vi "dirty_detector.vi"(10 "dirty ROI":T1(array[cluster]), 11 "pixel2mil":dbl) -> (3 "area":dbl)   [LabVIEW 2017]
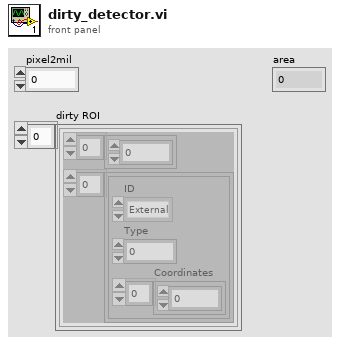
[diagram p1: front panel]
types:
  T1 = cluster{dbl[], cluster{"ID":enum32{"External", "Internal"}, "Type":u32, "Coordinates":i32[]}[]}[]
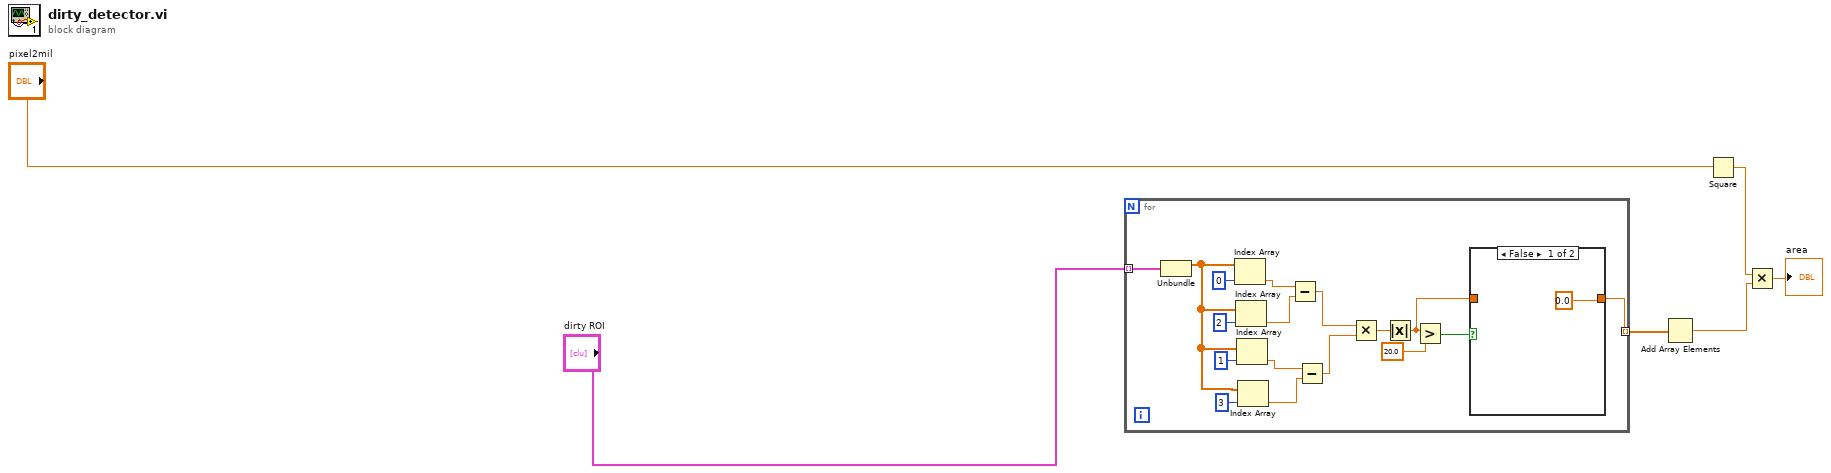
[diagram p0: block diagram]
diagram:
  n1 = for {
    tunnel: "dirty ROI" -> [w23] mode=indexing
    tunnel: [w8] -> w1 mode=indexing
    n2 = Unbundle(w23) -> (w18:dbl[])  [unwired: 1 out]
    n3 = Index Array(array=w18, index=0) -> (element=w17:dbl)
    n4 = Index Array(array=w18, index=2) -> (element=w16:dbl)
    n5 = Index Array(array=w18, index=1) -> (element=w15:dbl)
    n6 = Index Array(array=w18, index=3) -> (element=w14:dbl)
    n7 = Subtract(x=w17, y=w16) -> (x-y=w13:dbl)
    n8 = Subtract(x=w15, y=w14) -> (x-y=w12:dbl)
    n9 = Multiply(x=w13, y=w12) -> (x*y=w11:dbl)
    n10 = Absolute Value(x=w11) -> (abs(x)=w7:dbl)
    n11 = Greater?(x=w7, y=20.0) -> (0:w9:bool)
    n12 = case shown="False" w9 {
      tunnel: [0.0 ("y") w25] -> w8
      tunnel: w7 -> [_ w25]
      frame False {
      }
      frame True {
      }
    }
  }
  n13 = Add Array Elements(numeric array=w1) -> (sum=w5:dbl)
  n14 = Square(x="pixel2mil") -> (x^2=w4:dbl)
  n15 = Multiply(x=w4, y=w5) -> (x*y=→"area":dbl)
